vi "Scaling Exponent to Units.vi"(1 "Units":string, 3 "Scaling Exponent":dbl) -> (0 "Combined Units":string)   [LabVIEW 2020, in "GUCalibration2.lvlib"]
uses:
  GUCalibration2.lvlib
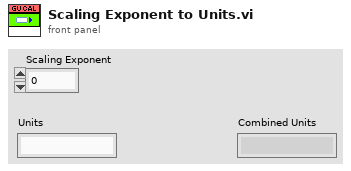
[diagram p1: front panel]
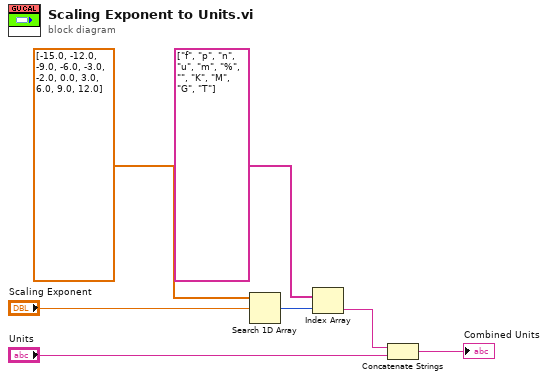
[diagram p0: block diagram]
diagram:
  n1 = Search 1D Array(1D array=dbl[] [-15.0, -12.0, -9.0, -6.0, -3.0, -2.0, 0.0, 3.0, 6.0, 9.0, 12.0] ("Strings []"), element="Scaling Exponent") -> (index of element=w5:i32)  [unwired: 1 in]
  n2 = Index Array(array=string[] ["f", "p", "n", "u", "m", "%", "", "K", "M", "G", "T"] ("Strings []"), index=w5) -> (element=w3:string)
  n3 = Concatenate Strings(w3, "Units") -> (→"Combined Units":string)
